vi "Resolve Referential Element.vi"(8 "error in":errorcluster, 10 "SNAME":string, 11 "Tree In":refnum<class "Tree.lvclass">) -> (0 "error out":errorcluster, 2 "Geometric":refnum<class "Geometric.lvclass">[](array[class]), 3 "Tree Out":refnum<class "Tree.lvclass">)   [LabVIEW 2019, in "ParseGDSII.lvclass"]
uses:
  ParseGDSII.lvclass
  Tree/Tree.lvclass
  Elements/Geometric.lvclass
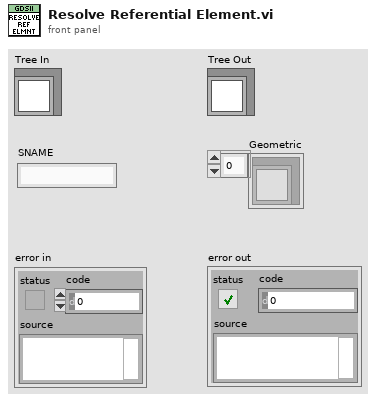
[diagram p1: front panel]
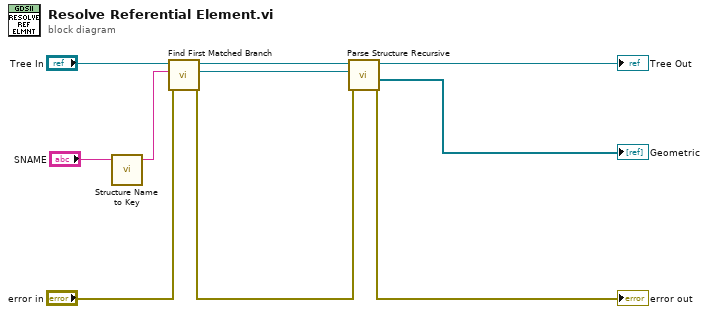
[diagram p0: block diagram]
diagram:
  n1 = call "Structure Name to Key.vi"("Name"="SNAME") -> ("Key"=w8:string)  [unwired: 4 in]
  n2 = call "Find First Matched Branch.vi"("error in"="error in", "Branch Name Exact"=w8, "Tree in"="Tree In") -> ("error out"=w3:errorcluster, "Matched Branch"=w4:refnum<class "Tree.lvclass">, "Tree out"=w6:refnum<class "Tree.lvclass">)  [unwired: 5 in, 1 out]
  n3 = call "Parse Structure Recursive.vi"("error in"=w3, "Structure In"=w4, "Tree In"=w6) -> ("error out"=→"error out":errorcluster, "Geometric"=→"Geometric":refnum<class "Geometric.lvclass">[], "Tree Out"=→"Tree Out":refnum<class "Tree.lvclass">)  [unwired: 5 in, 1 out]
